vi "test_libssh2_channel_eof.vi"() -> ()   [LabVIEW 2017, in "integration_tests.lvlib"]
uses:
  integration_tests.lvlib
  libssh2/libssh2_channel_open_ex.vi
  libssh2/libssh2_channel_process_startup.vi
  libssh2/libssh2_channel_read_ex.vi
  support/support.lvlib
  libssh2/libssh2.lvlib
  <vilib>/PNR/Transparent Assertions/Transparent Assertions/Transparent Assertions.lvlib
panel:
  out "error out":errorcluster
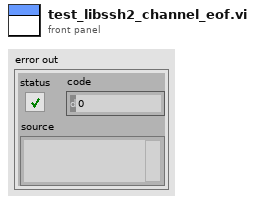
[diagram p1: front panel]
types:
  T1 = typedef "libssh2.lvlib/Session Refnum.ctl" = refnum<k1>
  T2 = typedef "libssh2.lvlib/Channel Refnum.ctl" = refnum<k1>
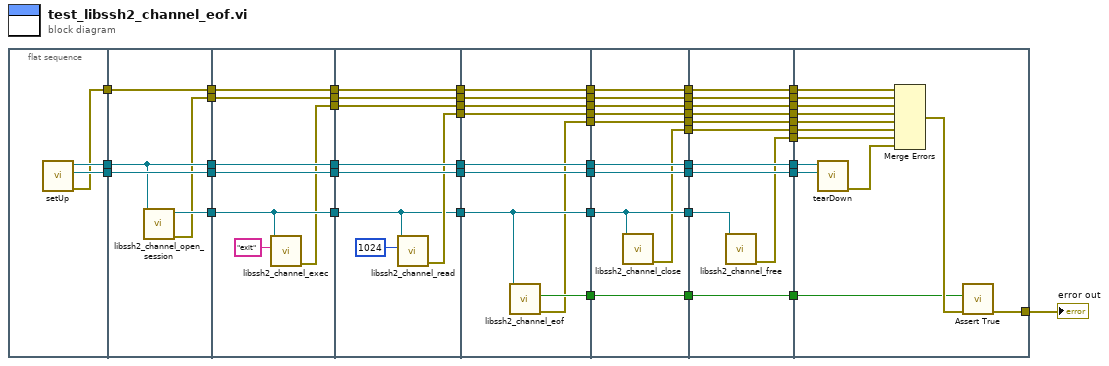
[diagram p0: block diagram]
diagram:
  n1 = flat-sequence {
    tunnel: [w54] -> w51
    tunnel: [w53] -> w50
    tunnel: [w52] -> w49
    tunnel: w51 -> [w58]
    tunnel: w50 -> [w59]
    tunnel: [w58] -> w37
    tunnel: [w59] -> w36
    tunnel: [w57] -> w35
    tunnel: w49 -> [w56]
    tunnel: [w56] -> w34
    tunnel: [w55] -> w33
    tunnel: w37 -> [w66]
    tunnel: [w66] -> w28
    tunnel: w36 -> [w65]
    tunnel: [w65] -> w27
    tunnel: w35 -> [w62]
    tunnel: [w62] -> w26
    tunnel: w34 -> [w64]
    tunnel: [w64] -> w25
    tunnel: w33 -> [w61]
    tunnel: [w61] -> w24
    tunnel: [w60] -> w23
    tunnel: w28 -> [w74]
    tunnel: [w74] -> w20
    tunnel: w27 -> [w73]
    tunnel: [w73] -> w18
    tunnel: w26 -> [w67]
    tunnel: [w67] -> w16
    tunnel: w25 -> [w72]
    tunnel: [w72] -> w14
    tunnel: w24 -> [w71]
    tunnel: [w71] -> w12
    tunnel: w23 -> [w70]
    tunnel: [w70] -> w10
    tunnel: [w68] -> w8
    tunnel: w20 -> [w83]
    tunnel: [w83] -> w19
    tunnel: w18 -> [w82]
    tunnel: [w82] -> w17
    tunnel: w16 -> [w77]
    tunnel: [w77] -> w15
    tunnel: w14 -> [w81]
    tunnel: [w81] -> w13
    tunnel: w12 -> [w80]
    tunnel: [w80] -> w11
    tunnel: w10 -> [w79]
    tunnel: [w79] -> w9
    tunnel: w8 -> [w78]
    tunnel: [w78] -> w7
    tunnel: [w76] -> w4
    tunnel: [w75] -> w3
    tunnel: w19 -> [w93]
    tunnel: w17 -> [w92]
    tunnel: w15 -> [w91]
    tunnel: [w93] -> w48
    tunnel: [w92] -> w47
    tunnel: [w91] -> w46
    tunnel: [w90] -> w45
    tunnel: w13 -> [w89]
    tunnel: [w89] -> w44
    tunnel: w11 -> [w88]
    tunnel: [w88] -> w32
    tunnel: w9 -> [w87]
    tunnel: [w87] -> w30
    tunnel: w7 -> [w86]
    tunnel: [w86] -> w22
    tunnel: [w85] -> w5
    tunnel: w4 -> [w85]
    tunnel: w3 -> [w84]
    tunnel: [w84] -> w2
    tunnel: w48 -> [w104]
    tunnel: w47 -> [w103]
    tunnel: w46 -> [w102]
    tunnel: [w104] -> w43
    tunnel: [w103] -> w42
    tunnel: [w101] -> w41
    tunnel: w45 -> [w100]
    tunnel: [w100] -> w40
    tunnel: w44 -> [w99]
    tunnel: [w99] -> w39
    tunnel: w32 -> [w98]
    tunnel: [w98] -> w31
    tunnel: w30 -> [w97]
    tunnel: [w97] -> w29
    tunnel: w22 -> [w96]
    tunnel: [w96] -> w21
    tunnel: [w95] -> w6
    tunnel: w5 -> [w95]
    tunnel: w2 -> [w94]
    tunnel: [w94] -> w1
    tunnel: w43 -> [w117]
    tunnel: w42 -> [w116]
    tunnel: [w115] -> w38
    tunnel: w41 -> [w113]
    tunnel: w40 -> [w112]
    tunnel: w39 -> [w111]
    tunnel: w31 -> [w109]
    tunnel: w29 -> [w108]
    tunnel: w21 -> [w107]
    tunnel: w6 -> [w106]
    tunnel: w1 -> [w105]
    frame #0 {
      n2 = call "setUp.vi"() -> ("error out"=w52:errorcluster, "connection ID"=w53:refnum<k5>, "session"=w54:T1)  [unwired: 9 in]
    }
    frame #1 {
      n3 = call "libssh2_channel_open_session.vi"("session"=w58) -> ("error out"=w55:errorcluster, "channel"=w57:T2)  [unwired: 9 in]
    }
    frame #2 {
      n4 = call "libssh2_channel_exec.vi"("command"="exit", "channel"=w62) -> ("error out"=w60:errorcluster)  [unwired: 9 in]
    }
    frame #3 {
      n5 = call "libssh2_channel_read.vi"("buffer length"=1024, "channel"=w67) -> ("error out"=w68:errorcluster)  [unwired: 8 in, 1 out]
    }
    frame #4 {
      n6 = call "libssh2_channel_eof.vi"("channel"=w77) -> ("error out"=w75:errorcluster, "eof"=w76:bool)  [unwired: 9 in]
    }
    frame #5 {
      n7 = call "libssh2_channel_close.vi"("channel"=w91) -> ("error out"=w90:errorcluster)  [unwired: 10 in]
    }
    frame #6 {
      n8 = call "libssh2_channel_free.vi"("channel"=w102) -> ("error out"=w101:errorcluster)  [unwired: 10 in]
    }
    frame #7 {
      n9 = call "tearDown.vi"("connection ID"=w116, "session"=w117) -> ("error out"=w114:errorcluster)  [unwired: 9 in]
      n10 = Merge Errors(w111, w109, w108, w107, w105, w112, w113, w114) -> (w110:errorcluster)
      n11 = call <vilib>:"Assert True.vi"("error in (no error)"=w110, "Condition"=w106) -> ("error out"=w115:errorcluster)  [unwired: 9 in]
    }
  }
  "error out" <- w38
